vi "Close.vi"(8 "error in (no error)":errorcluster, 11 "TD in":refnum<class "Test Device.lvclass">) -> (0 "error out":errorcluster)   [LabVIEW 2015, in "Test Device.lvclass"]
uses:
  Test Device.lvclass
  <vilib>/plasmapper/PL BlackBox Modbus CLient/PL BlackBox Modbus Client.lvclass
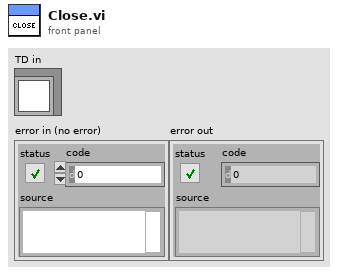
[diagram p1: front panel]
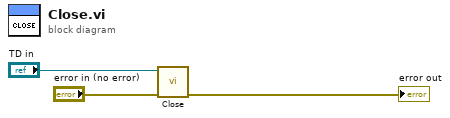
[diagram p0: block diagram]
diagram:
  n1 = call-parent "Close.vi"("error in (no error)"="error in (no error)", "PLBB in"="TD in") -> ("error out"=→"error out":errorcluster)  [unwired: 9 in]
